vi "E8267D VisaRW.vi"(4 "Délais (0 ms)":u32, 5 "Lecture?(T)":bool=TRUE, 6 "error in (no error)":errorcluster, 7 "Nbcaract":u32=100 caption="Nombre de \ncaractères à lire", 8 "Close(F)":bool, 9 "ChaineCom":string caption="Chaîne de commande", 10 "VISA Rsrc":refnum<visa-resource-name>="GPIB0::12::INSTR") -> (0 "error out":errorcluster, 1 "Count out":u32=44 caption="Nombre de caractères lus", 2 "ChaineRep":string caption="Chaîne de réponse", 3 "VISA Rsrc Out":refnum<visa-resource-name>="GPIB0::12::INSTR")   [LabVIEW 2019]
doc: "Ce VI envoie des commande d'écriture et de lecture VISA à l'appareil GPIB. Il permet de ne pas séparer un question de sa réponse. Pour que cela fonctionne toute lecture d'un instrument doit se faire par ce VI."
panel:
  in  "EOS (Aucun)":string
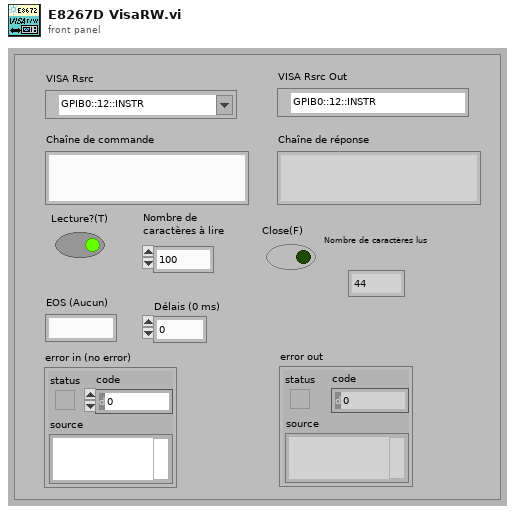
[diagram p1: front panel]
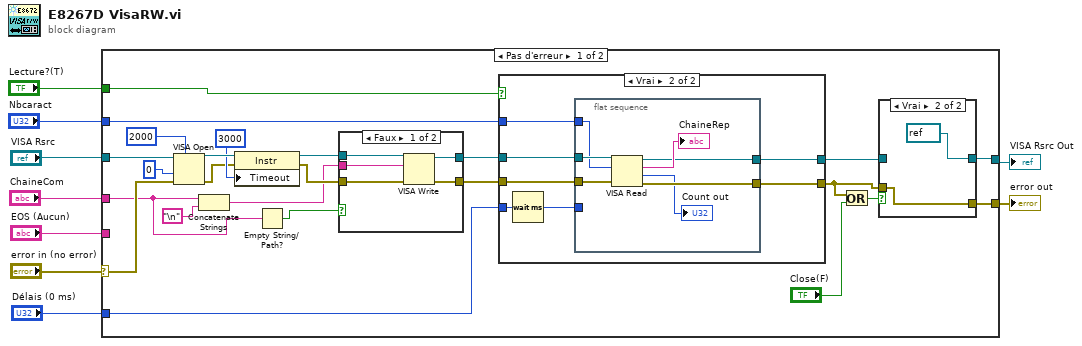
[diagram p0: block diagram]
diagram:
  n1 = case shown="Pas d'erreur" "error in (no error)" {
    selector: "error in (no error)" -> [w27 w62]
    tunnel: "VISA Rsrc" -> [w33 w61]
    tunnel: [w22 w61] -> w1
    tunnel: "ChaineCom" -> [w10 _]
    tunnel: "EOS (Aucun)" -> [_ _]
    tunnel: "Délais (0 ms)" -> [w30 _]
    tunnel: "Nbcaract" -> [w29 _]
    tunnel: "Lecture?(T)" -> [w28 _]
    tunnel: [w24 w62] -> w3
    frame No Error {
      n2 = VISA Open(timeout (0)=u32 2000 ("Timeout de VISA Open (0)"), access mode=u32 0, error in (no error)=w27, VISA resource name=w33) -> (VISA resource name=w20:refnum<visa-resource-name>, error out=w18:errorcluster)  [unwired: 1 in]
      n3 = Concatenate Strings(w10, "\n") -> (w13:string)
      n4 = property class="Instr"(reference=w20, error in=w18, "Timeout"=u32 3000 ("General Settings:Timeout Value")) -> (reference out=w21:refnum<visa-resource-name>, error out=w17:errorcluster)
      n5 = Empty String/Path?(string/path=w10) -> (empty?=w12:bool)
      n6 = case shown="Faux" w12 {
        tunnel: w13 -> [w38 _]
        tunnel: [w37 w40] -> w32
        tunnel: [w36 w39] -> w31
        tunnel: w21 -> [w35 w40]
        tunnel: w17 -> [w34 w39]
        frame False {
          n7 = VISA Write(VISA resource name=w35, write buffer=w38, error in (no error)=w34) -> (VISA resource name out=w37:refnum<visa-resource-name>, error out=w36:errorcluster)  [unwired: 1 out]
        }
        frame True {
        }
      }
      n8 = case shown="Vrai" w28 {
        tunnel: w32 -> [w46 w53]
        tunnel: [w46 w52] -> w23
        tunnel: w31 -> [w45 w51]
        tunnel: [w45 w50] -> w14
        tunnel: w29 -> [_ w49]
        tunnel: w30 -> [_ w48]
        frame False {
        }
        frame True {
          n9 = Wait (ms)(milliseconds to wait=w48) -> (millisecond timer value=w47:u32)
          n10 = flat-sequence {
            tunnel: [w56] -> w50
            tunnel: [w58] -> w52
            tunnel: w53 -> [w60]
            tunnel: w51 -> [w57]
            tunnel: w49 -> [w54]
            tunnel: w47 -> [_]
            frame #0 {
              n11 = VISA Read(VISA resource name=w60, byte count=w54, error in (no error)=w57) -> (VISA resource name out=w58:refnum<visa-resource-name>, read buffer=→"ChaineRep":string, return count=→"Count out":u32, error out=w56:errorcluster)
            }
          }
        }
      }
      n12 = Or(x=w14, y="Close(F)") -> (x .or. y?=w15:bool)
      n13 = case shown="Vrai" w15 {
        tunnel: [w42 refnum<visa-resource-name> refnum ("VISA resource name out")] -> w22
        tunnel: w23 -> [w42 _]
        tunnel: [w41 w43] -> w24
        tunnel: w14 -> [w41 w43]
        frame False {
        }
        frame True {
        }
      }
    }
    frame Error {
    }
  }
  "error out" <- w3
  "VISA Rsrc Out" <- w1
